vi "barf mt meat yield.vi"() -> ()   [LabVIEW 2014]
panel:
  in  "Galapalos?":bool
  out "Encounter Totals (%)":dbl[](array[numeric])
  out "Total Encounters":i32
  in  "stop":bool
  # "0:  Rollercoaster\n1:  Garbage Tourist\n2:  Angry Tourist\n3:  Horrible Tourist Family"
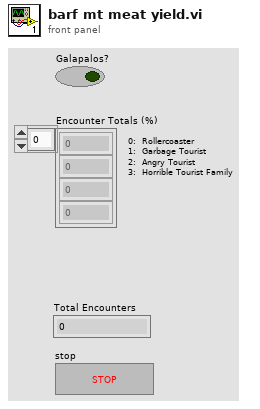
[diagram p1: front panel]
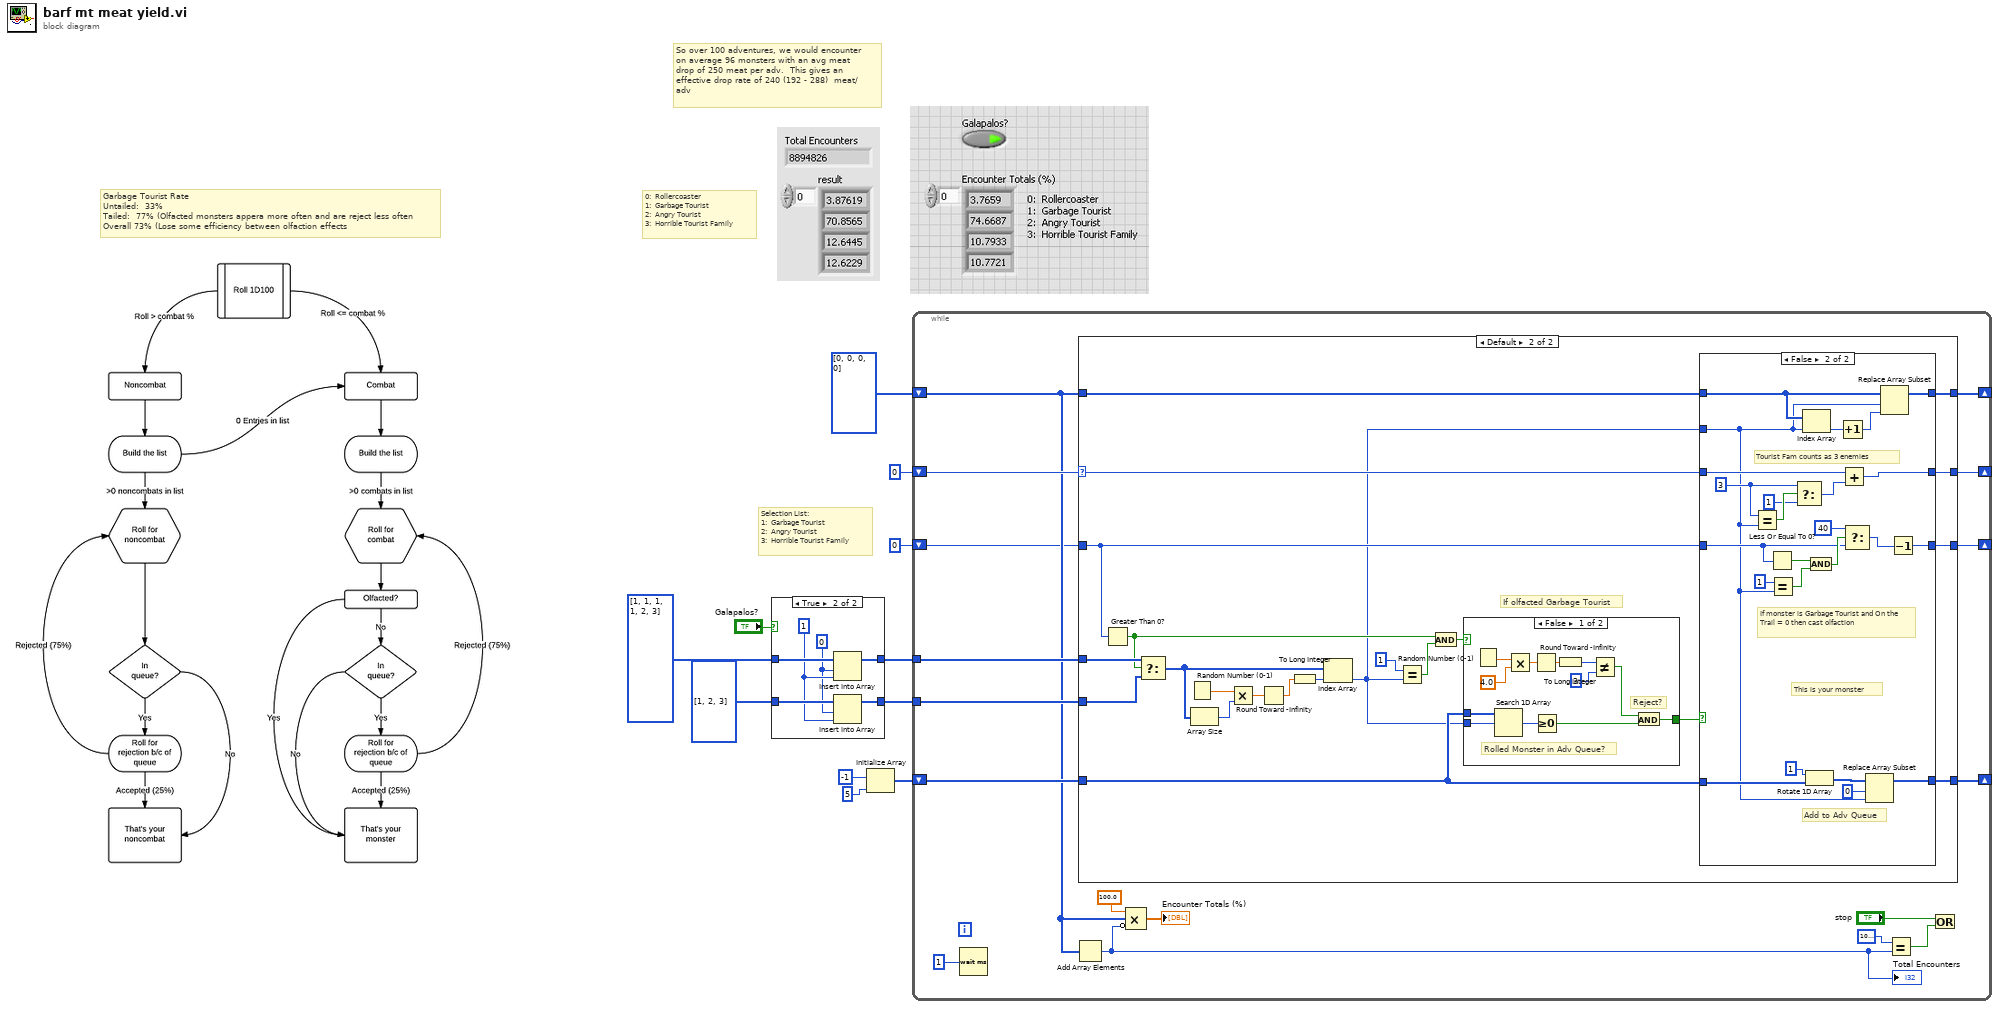
[diagram p0: block diagram]
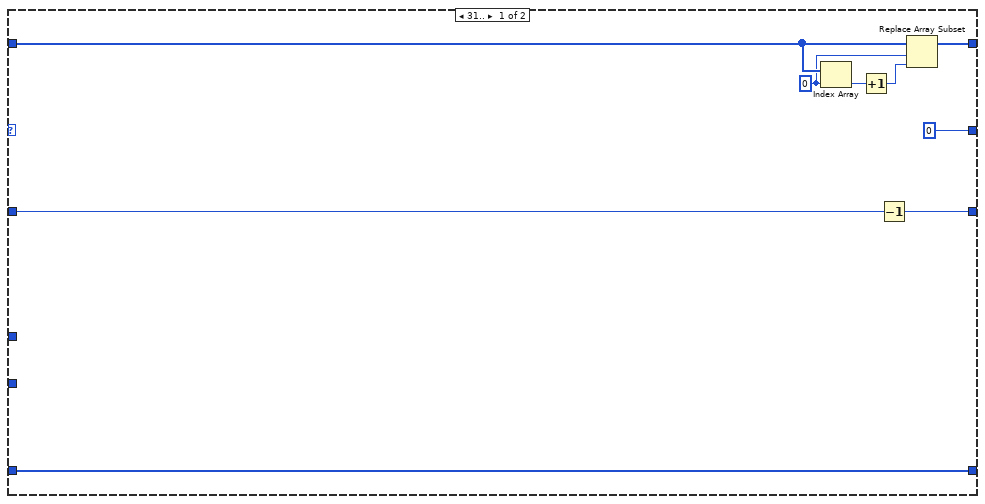
[diagram p3: hidden frame]
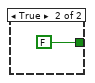
[diagram p5: hidden frame]
diagram:
  # "So over 100 adventures, we would encounter on average 96 monsters with an avg meat drop of 250 meat per adv.  This gives an effective drop rate of 240 (192 - 288)  meat/adv"
  # "0:  Rollercoaster\n1:  Garbage Tourist\n2:  Angry Tourist\n3:  Horrible Tourist Family"
  # "Garbage Tourist Rate\nUntailed:  33%\nTailed:  77% (Olfacted monsters appera more often and are reject less often\nOverall 73% (Lose some efficiency between olfaction effects"
  # "Selection List:\n1:  Garbage Tourist\n2:  Angry Tourist\n3:  Horrible Tourist Family"
  n1 = case shown="True" "Galapalos?" {
    tunnel: i32[] [1, 1, 1, 1, 2, 3] -> [w13 w19]
    tunnel: [w13 w18] -> w4
    tunnel: [w12 w17] -> w3
    tunnel: i32[] [1, 2, 3] -> [w12 w16]
    frame False {
    }
    frame True {
      w14 = 0 ("index")
      w15 = 1
      n2 = Insert Into Array(array=w19, index=w14, new element=w15) -> (w18:i32[])
      n3 = Insert Into Array(array=w16, index=w14, new element=w15) -> (w17:i32[])
    }
  }
  n4 = Initialize Array(-1, 5 ("dimension size")) -> (w9:i32[])
  n5 = while {
    tunnel: w4 -> [w31]
    shift-right: [w37] -> _
    shift-left: w9 -> [w29]
    tunnel: w3 -> [w30]
    shift-right: [w32] -> _
    shift-left: 0 -> [w20]
    shift-right: [w28] -> _
    shift-left: 0 -> [w27]
    shift-right: [w26] -> _
    shift-left: i32[] [0, 0, 0, 0] -> [w24]
    stop <- w36 stop-if-true
    n6 = Wait (ms)(milliseconds to wait=u32 1) -> ()  [unwired: 1 out]
    n7 = Add Array Elements(numeric array=w24) -> (sum=w23:i32)
    "Total Encounters" <- w23
    n8 = case shown="Default" w27 {
      selector: w27 -> [_ w50]
      tunnel: [w46 w64] -> w37
      tunnel: [w44 w62] -> w32
      tunnel: w20 -> [w43 w61]
      tunnel: w31 -> [_ w57]
      tunnel: w30 -> [_ w56]
      tunnel: w29 -> [w46 w52]
      tunnel: [0 w51] -> w28
      tunnel: w24 -> [w41 w49]
      tunnel: [w38 w48] -> w26
      frame 31.. {
        w40 = 0 ("index")
        n9 = Index Array(array=w41, index=w40) -> (element=w42:i32)
        n10 = Increment(x=w42) -> (x+1=w39:i32)
        n11 = Decrement(x=w43) -> (x-1=w44:i32)
        n12 = Replace Array Subset(array=w41, new element=w39, index=w40) -> (w38:i32[])
      }
      frame Default {
        # "If olfacted Garbage Tourist"
        n13 = Greater Than 0?(x=w61) -> (x > 0?=w53:bool)
        n14 = Select(t=w57, s=w53, f=w56) -> (s? t:f=w55:i32[])
        n15 = Random Number (0-1)() -> (number: 0 to 1=w68:dbl)
        n16 = Array Size(array=w55) -> (size(s)=w54:i32)
        n17 = Multiply(x=w68, y=w54) -> (x*y=w67:dbl)
        n18 = Round Toward -Infinity(1:w67) -> (0:w66:dbl)
        n19 = To Long Integer(number=w66) -> (32bit integer=w65:i32)
        n20 = Index Array(array=w55, index=w65) -> (element=w47:i32)
        n21 = Equal?(x=1 ("y"), y=w47) -> (x = y?=w59:bool)
        n22 = And(x=w53, y=w59) -> (x .and. y?=w58:bool)
        n23 = case shown="False" w58 {
          tunnel: [w101 FALSE] -> w63
          tunnel: w52 -> [w98 _]
          tunnel: w47 -> [w97 _]
          frame False {
            # "Rolled Monster in Adv Queue?"
            # "Reject?"
            n24 = Random Number (0-1)() -> (number: 0 to 1=w106:dbl)
            n25 = Search 1D Array(1D array=w98, element=w97) -> (index of element=w99:i32)  [unwired: 1 in]
            n26 = Multiply(x=w106, y=4.0) -> (x*y=w107:dbl)
            n27 = Round Toward -Infinity(1:w107) -> (0:w108:dbl)
            n28 = Greater Or Equal To 0?(x=w99) -> (x >= 0?=w100:bool)
            n29 = To Long Integer(number=w108) -> (32bit integer=w104:i32)
            n30 = Not Equal?(x=w104, y=3) -> (x != y?=w102:bool)
            n31 = And(x=w102, y=w100) -> (x .and. y?=w101:bool)
          }
          frame True {
          }
        }
        n32 = case shown="False" w63 {
          tunnel: [w72 w96] -> w64
          tunnel: w52 -> [w72 w92]
          tunnel: w61 -> [w71 w87]
          tunnel: [w71 w84] -> w62
          tunnel: w50 -> [w70 w83]
          tunnel: [w70 w78] -> w51
          tunnel: [w69 w75] -> w48
          tunnel: w49 -> [w69 w74]
          tunnel: w47 -> [_ w73]
          frame True {
            # "Rejected"
          }
          frame False {
            w81 = 3 ("x")
            # "Add to Adv Queue"
            # "If monster is Garbage Tourist and On the Trail = 0 then cast olfaction"
            # "Tourist Fam counts as 3 enemies"
            # "This is your monster"
            n33 = Equal?(x=w81, y=w73) -> (x = y?=w82:bool)
            n34 = Less Or Equal To 0?(x=w87) -> (x <= 0?=w89:bool)
            n35 = Equal?(x=1, y=w73) -> (x = y?=w90:bool)
            n36 = Select(t=w81, s=w82, f=1) -> (s? t:f=w80:i32)
            n37 = Index Array(array=w74, index=w73) -> (element=w77:i32)
            n38 = Rotate 1D Array(1:w92, 2:1 ("n")) -> (0:w93:i32[])
            n39 = And(x=w89, y=w90) -> (x .and. y?=w88:bool)
            n40 = Increment(x=w77) -> (x+1=w76:i32)
            n41 = Add(x=w83, y=w80) -> (x+y=w78:i32)
            n42 = Select(t=40, s=w88, f=w87) -> (s? t:f=w85:i32)
            n43 = Replace Array Subset(array=w93, new element=w73, index=0) -> (w96:i32[])
            n44 = Replace Array Subset(array=w74, new element=w76, index=w73) -> (w75:i32[])
            n45 = Decrement(x=w85) -> (x-1=w84:i32)
          }
        }
      }
    }
    n46 = Compound Arithmetic op=MULTIPLY(100.0, w24, invert w23) -> (→"Encounter Totals (%)":dbl[])
    n47 = Equal?(x=1000000, y=w23) -> (x = y?=w34:bool)
    n48 = Or(x="stop", y=w34) -> (x .or. y?=w36:bool)
  }
